vi "Drive Read Encoders.vi"(1 "Drive Info":T1) -> (0 "Drive Out":T1)   [LabVIEW 2013]
panel:
  out "Current angle (deg) 2":dbl(knob) scale=0.0..360.0
  out "Current angle (deg)":dbl(knob) scale=0.0..360.0
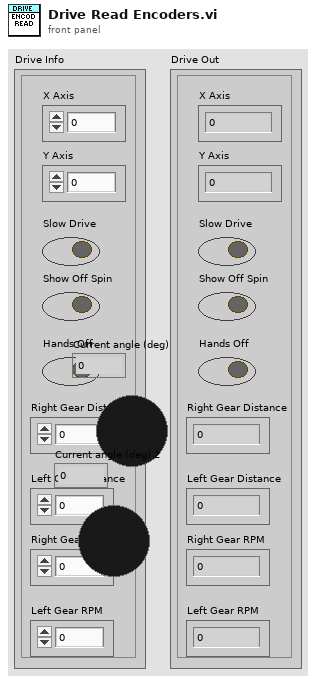
[diagram p1: front panel]
types:
  T1 = cluster{"X Axis":dbl, "Y Axis":dbl, "Slow Drive":bool, "Show Off Spin":bool, "Hands Off":bool, "Right Gear Distance":dbl, "Left Gear Distance ":dbl, "Right Gear RPM":dbl, "Left Gear RPM":dbl}
  T2 = typedef "WPI_EncoderDevRef.ctl" = cluster{"DevStatus":errorcluster, "EncoderIndex":T3, "CounterIndex":T4, "DistancePerCount":dbl, "Decoding Type":T5}
  T3 = typedef "FPGA_EncoderIdx.ctl" = enum8{"Enc 0", "Enc 1", "Enc 2", "Enc 3", "Invalid"}
  T4 = typedef "FPGA_CounterCtrSystemIndex.ctl" = enum8{"Ctr 0", "Ctr 1", "Ctr 2", "Ctr 3", "Ctr 4", "Ctr 5", "Ctr 6", "Ctr 7", "Invalid"}
  T5 = typedef "WPI_EncoderType.ctl" = enum16{"1x", "2x", "4x"}
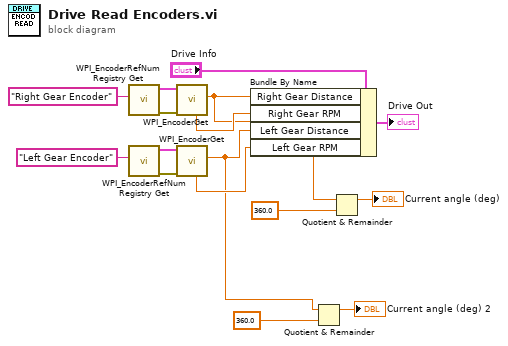
[diagram p0: block diagram]
diagram:
  n1 = call <vilib>:"WPI_EncoderRefNum Registry Get.vi"("refnum name"="Right Gear Encoder") -> ("error out"=w14:errorcluster, "EncoderDevRef"=w13:T2)  [unwired: 9 in]
  n2 = call <vilib>:"WPI_EncoderRefNum Registry Get.vi"("refnum name"="Left Gear Encoder") -> ("error out"=w12:errorcluster, "EncoderDevRef"=w11:T2)  [unwired: 9 in]
  n3 = call <vilib>:"WPI_EncoderGet.vi"("error in (no error)"=w14, "EncoderDevRef"=w13) -> ("Distance"=w4:dbl, "Rate"=w7:dbl)  [unwired: 4 in, 4 out]
  n4 = call <vilib>:"WPI_EncoderGet.vi"("error in (no error)"=w12, "EncoderDevRef"=w11) -> ("Distance"=w1:dbl, "Rate"=w8:dbl)  [unwired: 4 in, 4 out]
  n5 = Bundle By Name(cluster="Drive Info", "Right Gear Distance"=w4, "Right Gear RPM"=w7, "Left Gear Distance"=w1, "Left Gear RPM"=w8) -> (→"Drive Out":T1)
  n6 = Quotient & Remainder(x=w1, y=360.0) -> (x-y*floor(x/y)=→"Current angle (deg) 2":dbl)  [unwired: 1 out]
  n7 = Quotient & Remainder(x=w4, y=360.0) -> (x-y*floor(x/y)=→"Current angle (deg)":dbl)  [unwired: 1 out]
